vi "Get-latest-acquisition-stats.vi"(8 "error in (no error)":errorcluster, 11 "Data ref. in":refnum<data-value>) -> (0 "error out":errorcluster, 2 "Acq stats":T1, 3 "Data ref.":refnum<data-value>)   [LabVIEW 2013, in "CameraVision.lvlib" / "CV-Main.lvclass"]
uses:
  CV-Main.lvclass
  Acquisition/Acquisition-stats.ctl
  CV-Main.lvclass/CV-Main.ctl
  Read Acq stats.vi
  Acquisition/CV-Acquisition.lvclass
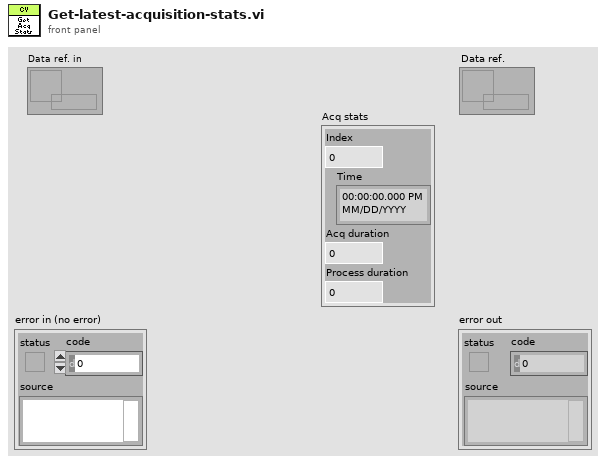
[diagram p1: front panel]
types:
  T1 = typedef "CameraVision.lvlib/CV-Acquisition.lvclass/Acquisition-stats.ctl" = cluster{"Index":i32, "Time":timestamp, "Acq duration":dbl, "Process duration":dbl}
  T2 = typedef "CameraVision.lvlib/Acquisition.lvclass/Acquisition-stats.ctl" = cluster{"Index":i32, "Time":timestamp, "Acq duration":dbl, "Process duration":dbl}
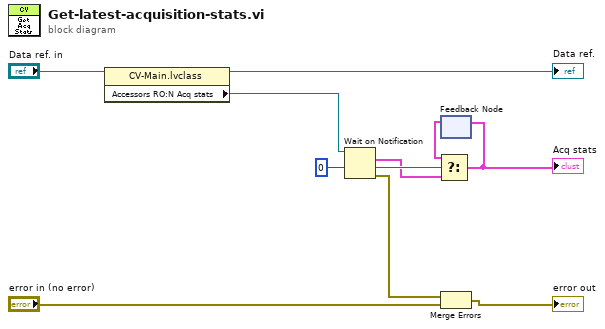
[diagram p0: block diagram]
diagram:
  n1 = property class="CV-Main.lvclass"(reference="Data ref. in") -> (reference out=→"Data ref.":refnum<data-value>, "Accessors RO:N Acq stats"=w6:refnum<notifier>)  [unwired: 1 in, 1 out]
  n2 = Wait on Notification(notifier=w6, timeout in ms (-1)=0) -> (notification=w2:T2, timed out?=w3:bool, error out=w1:errorcluster)  [unwired: 2 in, 1 out]
  n3 = feedback #1() -> (w4:T2)  [unwired: 1 in]
  n4 = Select(t=w4, s=w3, f=w2) -> (s? t:f=w7:T2)
  "Acq stats" <- w7
  n5 = feedback-in #1(w7) -> ()
  n6 = Merge Errors(w1, "error in (no error)") -> (→"error out":errorcluster)
